vi "VAR.vi"(0 "System no.":i32=1 min=1 max=4 step=1, 2 "Variable name":string, 3 "Value":string, 5 "error in":errorcluster) -> (19 "error out":errorcluster)   [LabVIEW 2020]
doc: "Sets a variable to a certain value. A variable is present in RAM only. See controller user manual for details regarding local and global variables.\n\nC-887, F-206, M-8X0: For GCS syntax version = GCS 2.0 or higher (Check with CSV?.vi. If CSV?.vi is not supported, syntax version is GCS 1.0).\n\nC-867, Mercury_GCS :"
panel:
  # "Sets a variable to a certain value. A variable is present in RAM only.\nSee controller User Manual for details regarding local and global variables."
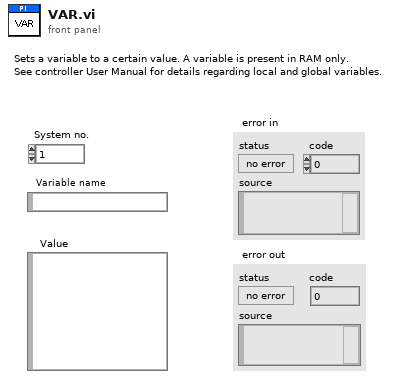
[diagram p1: front panel]
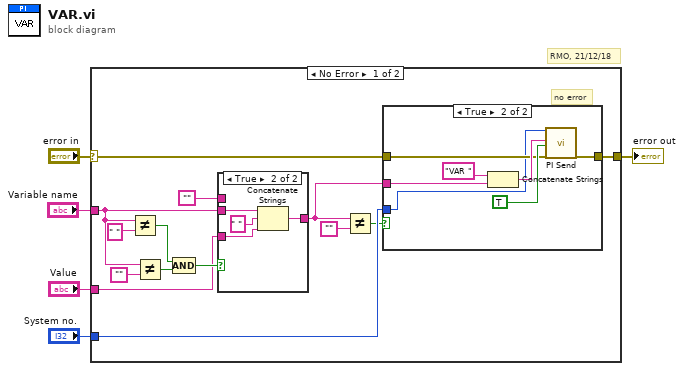
[diagram p0: block diagram]
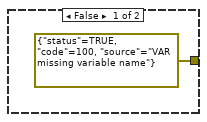
[diagram p3: hidden frame]
diagram:
  # "RMO, 21/12/18"
  n1 = case shown="No Error" "error in" {
    selector: "error in" -> [w6 w33]
    tunnel: "Variable name" -> [w9 _]
    tunnel: [w19 w33] -> w5
    tunnel: "Value" -> [w8 _]
    tunnel: "System no." -> [w18 _]
    frame No Error {
      # "no error"
      n2 = Not Equal?(x=w9, y=" ") -> (x != y?=w12:bool)
      n3 = Not Equal?(x=w9, y="") -> (x != y?=w11:bool)
      n4 = Compound Arithmetic op=AND(w12, w11) -> (w10:bool)
      n5 = case shown="True" w10 {
        tunnel: "" -> [w20 _]
        tunnel: w9 -> [_ w23]
        tunnel: [w20 w24] -> w16
        tunnel: w8 -> [_ w22]
        frame False {
        }
        frame True {
          n6 = Concatenate Strings(w23, " ", w22) -> (w24:string)
        }
      }
      n7 = Not Equal?(x=w16, y="") -> (x != y?=w15:bool)
      n8 = case shown="True" w15 {
        tunnel: w16 -> [_ w30]
        tunnel: w6 -> [_ w28]
        tunnel: w18 -> [_ w27]
        tunnel: [errorcluster {"status"=TRUE, "code"=100, "source"="VAR missing variable name"} ("error out") w26] -> w19
        frame False {
        }
        frame True {
          n9 = Concatenate Strings("VAR ", w30) -> (w29:string)
          n10 = call "PI Send.vi"("System no."=w27, "String to send"=w29, "Attach termination char.?"=TRUE ("Attach Linefeed?"), "error in"=w28) -> ("error out"=w26:errorcluster)  [unwired: 2 in, 13 out]
        }
      }
    }
    frame Error {
    }
  }
  "error out" <- w5
